vi "Find Sequencing Command Names.vi"(10 "project root path":path, 11 "TargetItem in":refnum<vi>) -> (2 "Paths":path[](array[path]), 3 "Command Info":T2(array[cluster]))   [LabVIEW 2025]
uses:
  <vilib>/picture/picture.llb/imagedata.ctl
  <vilib>/Utility/Data Type/NI_Data Type.lvlib
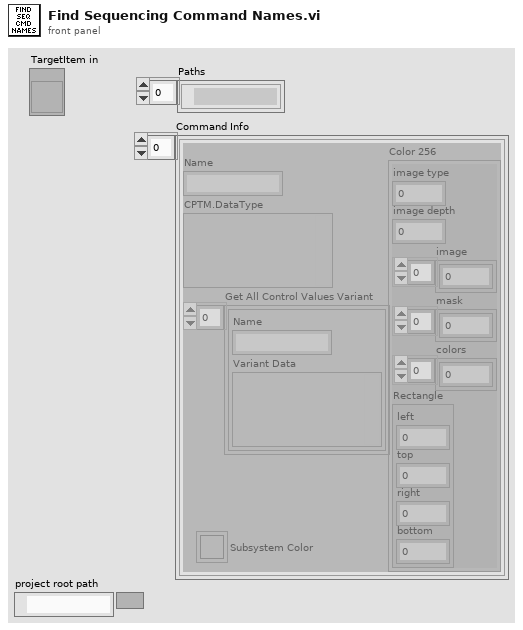
[diagram p1: front panel]
types:
  T1 = typedef "imagedata.ctl" = cluster{"image type":i32, "image depth":i32, "image":u8[], "mask":u8[], "colors":u32[], "Rectangle":cluster{"left":i16, "top":i16, "right":i16, "bottom":i16}}
  T2 = cluster{"Name":string, "CPTM.DataType":variant, "Get All Control Values Variant":cluster{"Name":string, "Variant Data":variant}[], "Color 256":T1, "Subsystem Color":u32}[]
  T3 = typedef "NI_Data Type.lvlib/Type Definition Info.ctl" = cluster{"Name":string, "Timestamp":u32}
  T4 = cluster{"Name":string, "CPTM.DataType":variant, "Get All Control Values Variant":cluster{"Name":string, "Variant Data":variant}[], "ImageData":T1, "Color Box":u32}
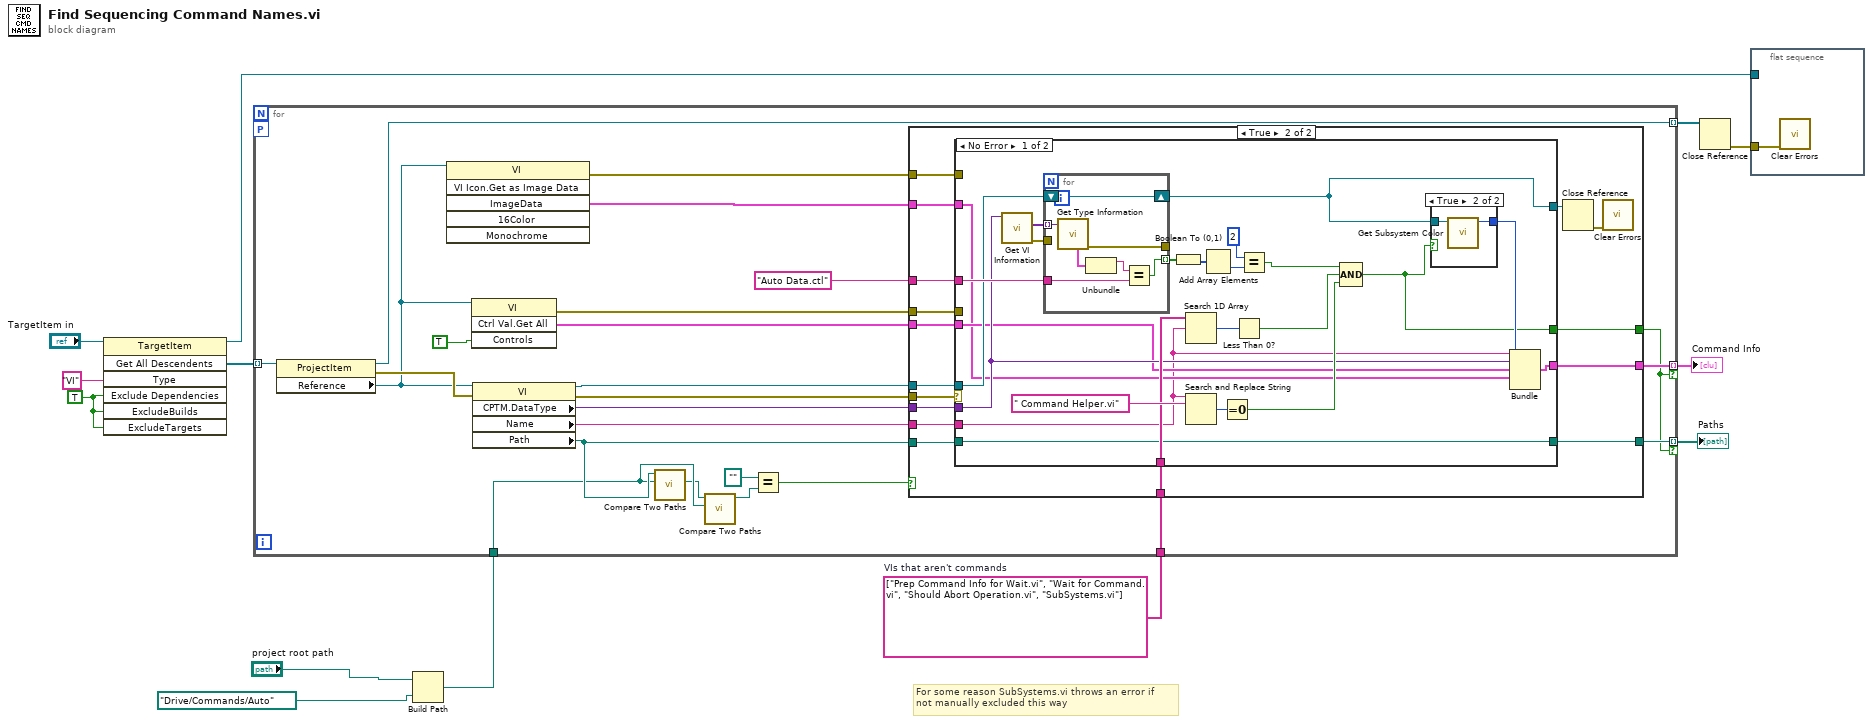
[diagram p0: block diagram]
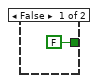
[diagram p2: hidden frame]
diagram:
  w10 = TRUE ("ExcludeDependencies")
  w8 = string[] ["Prep Command Info for Wait.vi", "Wait for Command.vi", "Should Abort Operation.vi", "SubSystems.vi"]  # VIs that aren't commands
  # "For some reason SubSystems.vi throws an error if \nnot manually excluded this way"
  n1 = invoke class="TargetItem" method="Get All Descendents"(reference="TargetItem in", "Type"="VI", "Exclude Dependencies"=w10, "ExcludeBuilds"=w10, "ExcludeTargets"=w10) -> (reference out=w4:refnum<vi>, "All Descendents"=w11:refnum<vi>[])  [unwired: 2 in, 5 out]
  n2 = Build Path(base path="project root path", name or relative path=path "Drive/Commands/Auto") -> (appended path=w2:path)
  n3 = for {
    tunnel: w11 -> [w37] mode=indexing
    tunnel: w8 -> [w35]
    tunnel: [w30] -> w12 mode=indexing if=w20
    tunnel: [w29] -> w13 mode=indexing if=w20
    tunnel: [w22] -> w5 mode=indexing
    tunnel: w2 -> [w18]
    workers-P: _ -> [_]
    n4 = property class="ProjectItem"(reference=w37) -> (reference out=w22:refnum<vi>, error out=w32:errorcluster, "Reference"=w25:refnum<vi>)  [unwired: 1 in]
    n5 = invoke class="VI" method="VI Icon.Get as Image Data"(reference=w25) -> (error out=w23:errorcluster, "ImageData"=w24:T1)  [unwired: 5 in, 4 out]
    n6 = invoke class="VI" method="Ctrl Val.Get All"(reference=w25, "Controls"=TRUE) -> (error out=w26:errorcluster, "Get All Control Values Variant"=w27:cluster{"Name":string, "Variant Data":variant}[])  [unwired: 2 in, 2 out]
    n7 = property class="VI"(reference=w25, error in=w32) -> (reference out=w21:refnum<vi>, error out=w31:errorcluster, "CPTM.DataType"=w34:variant, "Name"=w33:string, "Path"=w19:path)
    n8 = call <vilib>:"Compare Two Paths.vi"("Path 2"=w18, "Path 1"=w19) -> ("Common Path"=w16:path)  [unwired: 6 in, 3 out]
    n9 = call <vilib>:"Compare Two Paths.vi"("Path 2"=w18, "Path 1"=w16) -> ("Relative Path from 1 to 2"=w15:path)  [unwired: 6 in, 3 out]
    n10 = Equal?(x=path "", y=w15) -> (x = y?=w17:bool)
    n11 = case shown="True" w17 {
      tunnel: "Auto Data.ctl" ("Name") -> [_ w54]
      tunnel: w35 -> [_ w53]
      tunnel: w34 -> [_ w52]
      tunnel: w33 -> [_ w51]
      tunnel: w31 -> [_ w48]
      tunnel: [_ w47] -> w30
      tunnel: [_ w46] -> w29
      tunnel: w27 -> [_ w45]
      tunnel: w26 -> [_ w44]
      tunnel: w24 -> [_ w43]
      tunnel: w23 -> [_ w42]
      tunnel: w21 -> [_ w41]
      tunnel: [FALSE w40] -> w20
      tunnel: w19 -> [_ w39]
      frame False {
      }
      frame True {
        n12 = case shown="No Error" w48 {
          tunnel: w54 -> [w70 _]
          tunnel: w53 -> [w69 _]
          tunnel: w52 -> [w64 _]
          tunnel: w51 -> [w59 _]
          tunnel: [w61 w88] -> w49
          tunnel: w41 -> [w67 w88]
          tunnel: [w65 _] -> w47
          tunnel: w39 -> [w66 _]
          tunnel: [w66 _] -> w46
          tunnel: w45 -> [w63 _]
          tunnel: w44 -> [_ _]
          tunnel: w43 -> [w62 _]
          tunnel: w42 -> [_ _]
          tunnel: [w58 _] -> w40
          frame No Error {
            n13 = call <vilib>:"Get VI Information.vi"("variant"=w64) -> ("error out"=w73:errorcluster, "VI terminal types"=w72:variant[])  [unwired: 7 in, 2 out]
            n14 = for {
              tunnel: w70 -> [w87]
              tunnel: [w86] -> w71 mode=indexing
              tunnel: w72 -> [w84] mode=indexing
              tunnel: w73 -> [_]
              tunnel: [w83] -> _
              shift-right: [w85] -> w61
              shift-left: w67 -> [w85]
              n15 = call <vilib>:"Get Type Information.vi"("variant"=w84) -> ("error out"=w83:errorcluster, "type definition info"=w82:T3)  [unwired: 6 in, 3 out]
              n16 = Unbundle(w82) -> ("Name"=w81:string)  [unwired: 1 out]
              n17 = Equal?(x=w81, y=w87) -> (x = y?=w86:bool)
            }
            n18 = Boolean To (0,1)(Boolean=w71) -> (0, 1=w68:i16[])
            n19 = Search 1D Array(1D array=w69, element=w59) -> (index of element=w75:i32)  [unwired: 1 in]
            n20 = Search and Replace String(input string=w59, search string=" Command Helper.vi") -> (number of replacements=w77:i32)  [unwired: 6 in, 3 out]
            n21 = Add Array Elements(numeric array=w68) -> (sum=w57:i16)
            n22 = Equal To 0?(x=w77) -> (x = 0?=w78:bool)
            n23 = Less Than 0?(x=w75) -> (x < 0?=w76:bool)
            n24 = Equal?(x=2, y=w57) -> (x = y?=w55:bool)
            n25 = Compound Arithmetic op=AND(w55, w76, w78) -> (w58:bool)
            n26 = case shown="True" w58 {
              tunnel: w61 -> [_ w80]
              tunnel: [_ w79] -> w60
              frame False {
              }
              frame True {
                n27 = call "Get Subsystem Color.vi"("VI in"=w80) -> ("Color Box"=w79:u32)  [unwired: 10 in]
              }
            }
            n28 = Bundle("Name"=w59, "CPTM.DataType"=w64, "Get All Control Values Variant"=w63, "ImageData"=w62, "Color Box"=w60) -> (w65:T4)  [unwired: 1 in]
          }
          frame Error {
          }
        }
        n29 = Close Reference(reference=w49) -> (error out=w50:errorcluster)  [unwired: 1 in]
        n30 = call <vilib>:"Clear Errors.vi"("error in (no error)"=w50) -> ()  [unwired: 5 in, 2 out]
      }
    }
  }
  "Paths" <- w13
  "Command Info" <- w12
  n31 = Close Reference(reference=w5) -> (error out=w6:errorcluster)  [unwired: 1 in]
  n32 = flat-sequence {
    tunnel: w6 -> [w89]
    tunnel: w4 -> [_]
    frame #0 {
      n33 = call <vilib>:"Clear Errors.vi"("error in (no error)"=w89) -> ()  [unwired: 5 in, 2 out]
    }
  }
